vi "Encode Frame.vi"(8 "error in (no error)":errorcluster, 9 "payload":string, 11 "Ethernet Header":T1={"destination MAC address"={0, 0, 0, 0, 0, 0}, "source MAC address"={0, 0, 0, 0, 0, 0}, "Has VLAN Tag"=FALSE, "VLAN Tag"={"TPID"=33024, "priority"=0, "DEI"=FALSE, "VID"=0}, "Ethertype"=0} {"Ethertype" format="%.0x"; "VLAN Tag"."VID" format="%.0x"; "VLAN Tag"."TPID" format="%.0x"; "source MAC address"."?" format="%02x"; "source MAC address"."?" format="%02x"; "source MAC address"."?" format="%02x"; "source MAC address"."?" format="%02x"; "source MAC address"."?" format="%02x"; "source MAC address"."?" format="%02x"; "destination MAC address"."?" format="%02x"; "destination MAC address"."?" format="%02x"; "destination MAC address"."?" format="%02x"; "destination MAC address"."?" format="%02x"; "destination MAC address"."?" format="%02x"; "destination MAC address"."?" format="%02x"}) -> (0 "error out":errorcluster, 3 "frame data":u8[](array[numeric]))   [LabVIEW 2025, in "Automotive Ethernet Bus Monitor.lvclass"]
uses:
  Automotive Ethernet Bus Monitor.lvclass
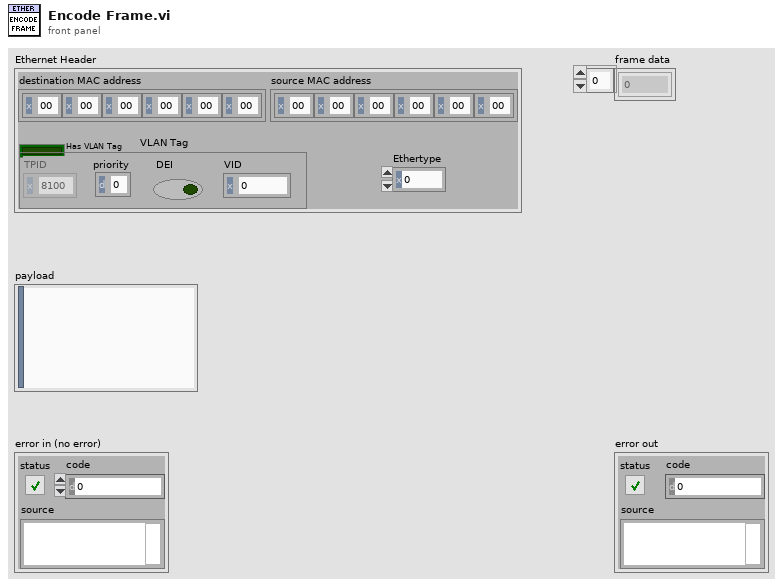
[diagram p1: front panel]
types:
  T1 = cluster{"destination MAC address":cluster{u8, u8, u8, u8, u8, u8}, "source MAC address":cluster{u8, u8, u8, u8, u8, u8}, "Has VLAN Tag":bool, "VLAN Tag":cluster{"TPID":u16, "priority":u8, "DEI":bool, "VID":u16}, "Ethertype":u16}
  T2 = cluster{"TPID":u16, "priority":u8, "DEI":bool, "VID":u16}
  T3 = cluster{"destination MAC address":cluster{u8, u8, u8, u8, u8, u8}, "source MAC address":cluster{u8, u8, u8, u8, u8, u8}}
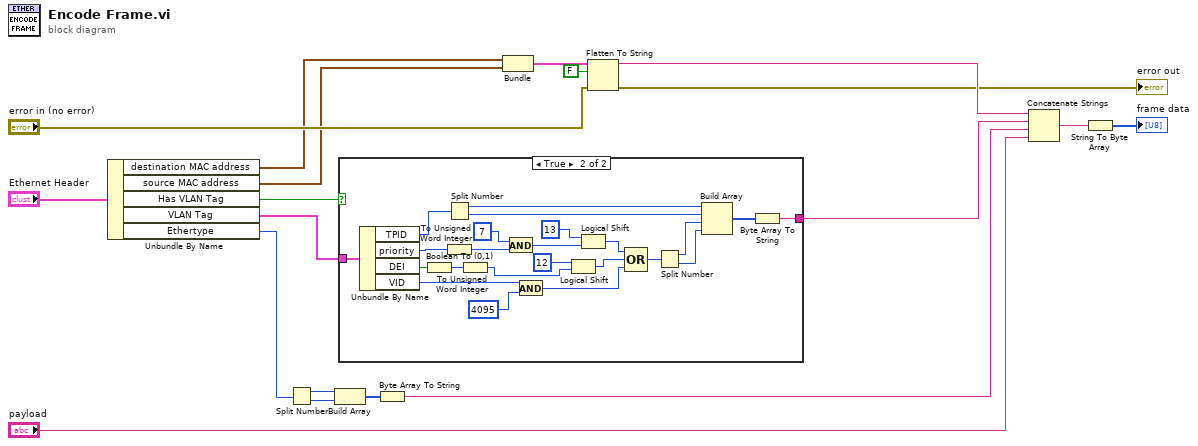
[diagram p0: block diagram]
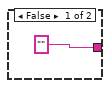
[diagram p2: hidden frame]
diagram:
  n1 = Unbundle By Name("Ethernet Header") -> ("destination MAC address"=w8:cluster{u8, u8, u8, u8, u8, u8}, "source MAC address"=w7:cluster{u8, u8, u8, u8, u8, u8}, "Has VLAN Tag"=w5:bool, "VLAN Tag"=w6:T2, "Ethertype"=w1:u16)
  n2 = Split Number(x=w1) -> (hi(x)=w14:u8, lo(x)=w13:u8)
  n3 = Build Array(w14, w13) -> (w12:u8[])
  n4 = case shown="True" w5 {
    tunnel: ["" ("string") w42] -> w15
    tunnel: w6 -> [_ w21]
    frame False {
    }
    frame True {
      n5 = Unbundle By Name(w21) -> ("TPID"=w41:u16, "priority"=w33:u8, "DEI"=w36:bool, "VID"=w38:u16)
      n6 = Boolean To (0,1)(Boolean=w36) -> (0, 1=w35:i16)
      n7 = To Unsigned Word Integer(number=w33) -> (unsigned 16bit integer=w32:u16)
      n8 = Split Number(x=w41) -> (hi(x)=w40:u8, lo(x)=w39:u8)
      n9 = To Unsigned Word Integer(number=w35) -> (unsigned 16bit integer=w29:u16)
      n10 = And(x=u16 7 ("y"), y=w32) -> (x .and. y?=w30:u16)
      n11 = And(x=w38, y=u16 4095) -> (x .and. y?=w27:u16)
      n12 = Logical Shift(y=i16 12, x=w29) -> (x << y=w26:u16)
      n13 = Logical Shift(y=i16 13, x=w30) -> (x << y=w25:u16)
      n14 = Compound Arithmetic op=OR(w25, w26, w27) -> (w24:u16)
      n15 = Split Number(x=w24) -> (hi(x)=w23:u8, lo(x)=w22:u8)
      n16 = Build Array(w40, w39, w23, w22) -> (w43:u8[])
      n17 = Byte Array To String(unsigned byte array=w43) -> (string=w42:string)
    }
  }
  n18 = Byte Array To String(unsigned byte array=w12) -> (string=w11:string)
  n19 = Bundle("destination MAC address"=w8, "source MAC address"=w7) -> (w19:T3)  [unwired: 1 in]
  n20 = Flatten To String(anything=w19, prepend array or string size? (T)=FALSE, error in (no error)="error in (no error)") -> (data string=w16:string, error out=→"error out":errorcluster)  [unwired: 1 in, 1 out]
  n21 = Concatenate Strings(w16, w15, w11, "payload") -> (w4:string)
  n22 = String To Byte Array(string=w4) -> (unsigned byte array=→"frame data":u8[])
